vi "GenerateMR.vi"(0 "String In":string) -> (1 "Motion Resource Out":refnum<k21>, 2 "number":u32 format="%x")   [LabVIEW 2011]
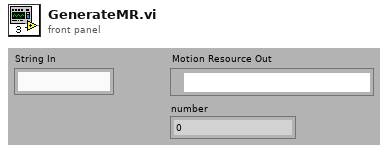
[diagram p1: front panel]
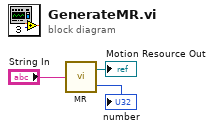
[diagram p0: block diagram]
diagram:
  n1 = call "MR.vi"("Motion Resource In"="String In") -> ("Motion Resource Out"=→"Motion Resource Out":refnum<k21>, "number"=→"number":u32)
